vi "BRig_RT_comm_tcp_write_RTwrite__RunState_Trial_end.vi"(11 "input_dataCurrent":u16[](array[numeric])) -> (2 "output_strCmd":string)   [LabVIEW 2014]
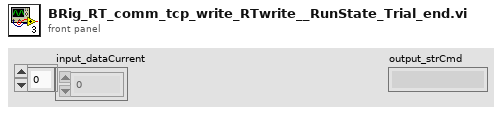
[diagram p1: front panel]
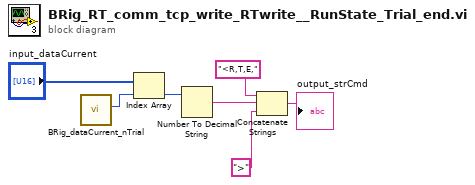
[diagram p0: block diagram]
diagram:
  n1 = call "BRig_dataCurrent_nTrial.vi"() -> ("output_nTrial"=w7:i32)  [unwired: 11 in]
  n2 = Index Array(array="input_dataCurrent", index=w7) -> (element=w6:u16)
  n3 = Number To Decimal String(number=w6) -> (decimal integer string=w5:string)  [unwired: 1 in]
  n4 = Concatenate Strings("<R,T,E," ("string"), w5, ">" ("string")) -> (→"output_strCmd":string)
